vi "Data Acquisition module.vi"(3 "PortName":string, 4 "Gas Presure":dbl[unit]=80000.0 min=80000.0 max=120000.0, 5 "Run":bool=TRUE) -> (0 "Pre Evaporation Water Flow Detected by sensor":dbl[unit], 1 "Flow Evaporation Water Detected by sensor":dbl[unit], 2 "MFRHA\nMass Flow Rate of Humid Air \nof Input(Kg/s)":dbl[unit])   [LabVIEW 2018]
panel:
  out "Temp Evaporator Water  Out":dbl[unit]
  out "Voltage Level FlowMeter Air ZeroFlow":dbl
  out "Voltage Level FlowMeter.Pre.EVA Ziro Flow Water":dbl
  out "Voltage Level FlowMeter.EVA ZiroFlow Water":dbl
  out "Humidity 3rd":dbl
  out "Humidity Evaporator IN":dbl
  out "Humidity Evaporator OUT":dbl
  out "Temp 3rd Air":dbl[unit]
  out "Temp Evaporator Air IN":dbl[unit]
  out "Temp Evaporator Air OUT":dbl[unit]
  out "Voltage Level Flowmeter Air":dbl
  out "Voltage Level Flowmeter.Pre Eva Water":dbl
  out "Voltage Level Flowmeter.EVA Water":dbl
  out "Temp water  Series 2":dbl[unit]
  out "Temp Pre Eva  Water OUT":dbl[unit]
  out "Temp Pre Eva water IN":dbl[unit]
  out "Temp Evaporator Water IN":dbl[unit]
  out "SHT/H":dbl[](array[numeric])
  out "SHT/T":dbl[unit][](array[numeric])
  out "EEP":dbl[](array[numeric])
  out "MPX":dbl[](array[numeric])
  out "DS18b20":dbl[unit][](array[numeric])
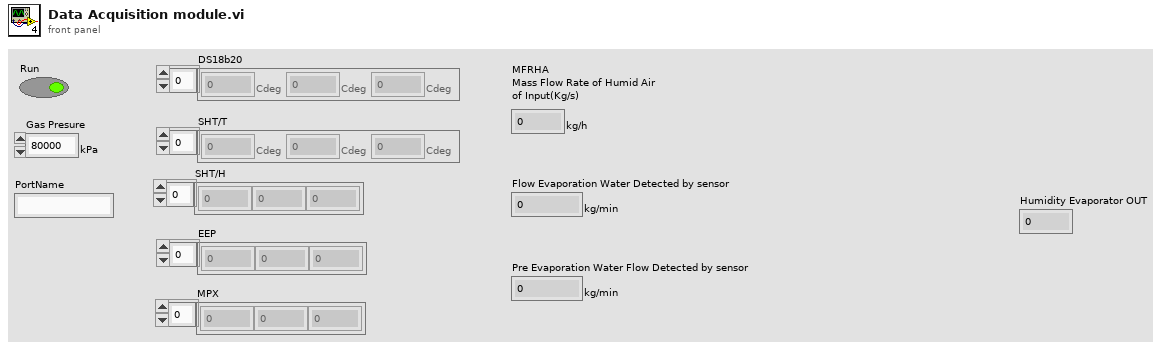
[diagram p1: front panel]
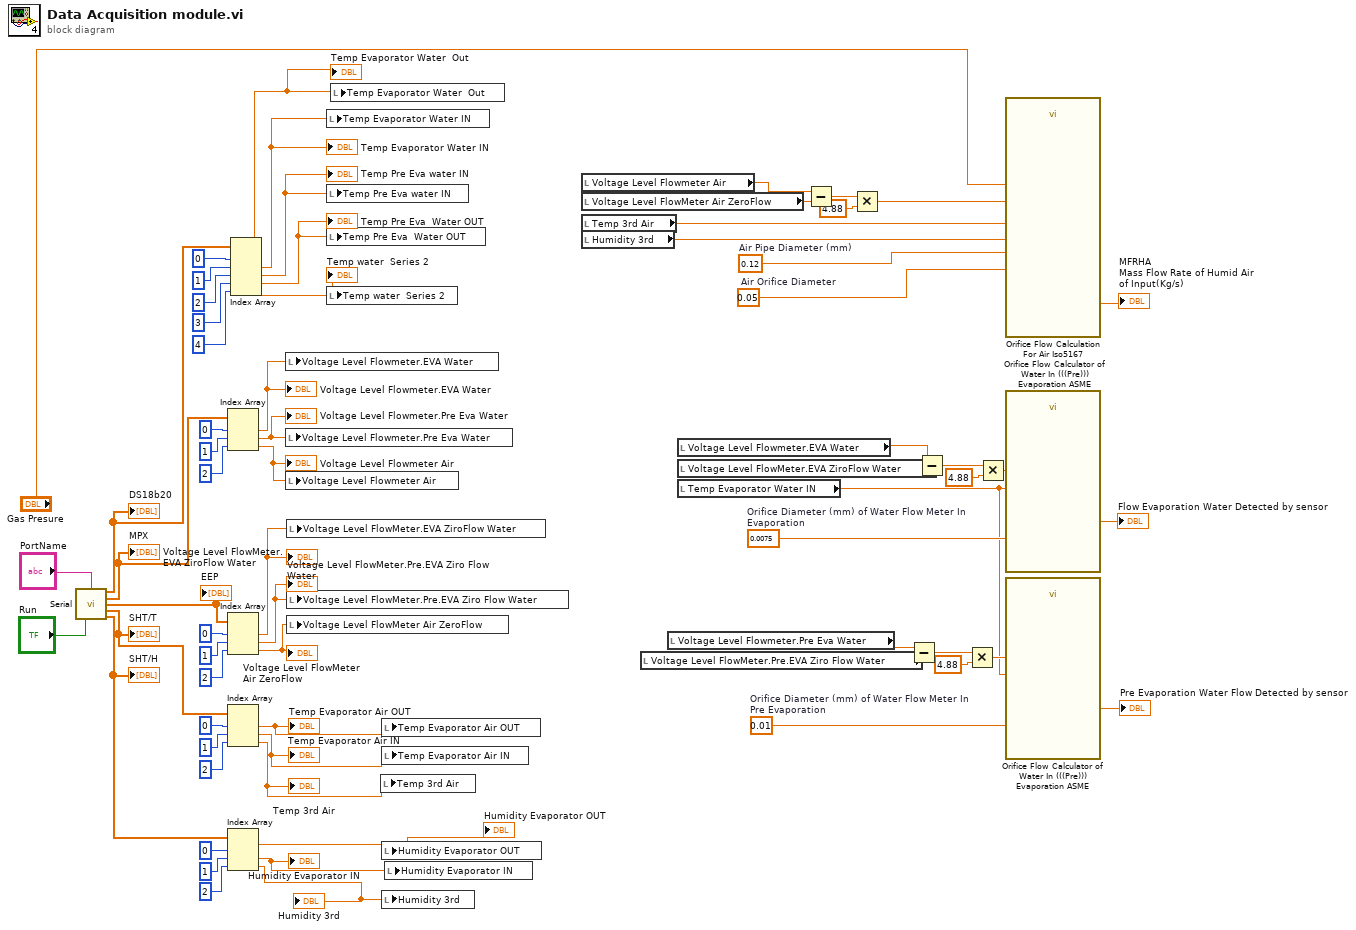
[diagram p0: block diagram]
diagram:
  w55 = dbl[unit] 0.0075  # Orifice Diameter (mm) of Water Flow Meter In Evaporation
  w66 = dbl[unit] 0.12  # Air Pipe Diameter (mm)
  w15 = dbl[unit] 0.05  # Air Orifice Diameter
  w59 = dbl[unit] 0.01  # Orifice Diameter (mm) of Water Flow Meter In Pre Evaporation
  n1 = call "Serial.vi"("PortName"="PortName", "Run"="Run") -> ("DS18b20"=w54:dbl[unit][], "MPX"=w48:dbl[], "EEP"=w33:dbl[], "SHT/H"=w44:dbl[unit][], "SHT/T"=w34:dbl[])  [unwired: 4 in, 5 out]
  "DS18b20" <- w54
  "MPX" <- w48
  "EEP" <- w33
  "SHT/T" <- w44
  "SHT/H" <- w34
  n2 = Index Array(array=w48, index #1=0 ("index"), index #2=1 ("index"), index #3=2 ("index")) -> (element #1=w29:dbl, element #2=w28:dbl, element #3=w18:dbl)
  "Voltage Level Flowmeter.EVA Water" <- w29
  "Voltage Level Flowmeter.Pre Eva Water" <- w28
  "Voltage Level Flowmeter Air" <- w18
  n3 = Index Array(array=w33, index #1=0 ("index"), index #2=1 ("index"), index #3=2 ("index")) -> (element #1=w27:dbl, element #2=w26:dbl, element #3=w25:dbl)
  "Voltage Level FlowMeter.EVA ZiroFlow Water" <- w27
  "Voltage Level FlowMeter.Pre.EVA Ziro Flow Water" <- w26
  "Voltage Level FlowMeter Air ZeroFlow" <- w25
  n4 = Index Array(array=w44, index #1=0 ("index"), index #2=1 ("index"), index #3=2 ("index")) -> (element #1=w23:dbl[unit], element #2=w24:dbl[unit], element #3=w22:dbl[unit])
  "Temp Evaporator Air OUT" <- w23
  "Temp Evaporator Air IN" <- w24
  "Temp 3rd Air" <- w22
  n5 = Index Array(array=w34, index #1=0 ("index"), index #2=1 ("index"), index #3=2 ("index")) -> (element #1=w20:dbl, element #2=w6:dbl, element #3=w21:dbl)
  "Humidity Evaporator OUT" <- w20
  "Humidity Evaporator IN" <- w6
  "Humidity 3rd" <- w21
  n6 = Index Array(array=w54, index #1=0 ("index"), index #2=1 ("index"), index #3=2 ("index"), index #4=3 ("index"), index #5=4 ("index")) -> (element #1=w3:dbl[unit], element #2=w9:dbl[unit], element #3=w37:dbl[unit], element #4=w36:dbl[unit], element #5=w35:dbl[unit])
  "Temp Evaporator Water IN" <- w9
  "Temp Pre Eva water IN" <- w37
  "Temp Pre Eva  Water OUT" <- w36
  "Temp water  Series 2" <- w35
  "Temp Evaporator Water  Out" <- w3
  n7 = local write "Voltage Level Flowmeter.EVA Water"(w29) -> ()
  n8 = local write "Voltage Level Flowmeter.Pre Eva Water"(w28) -> ()
  n9 = local write "Voltage Level Flowmeter Air"(w18) -> ()
  n10 = local write "Voltage Level FlowMeter.EVA ZiroFlow Water"(w27) -> ()
  n11 = local write "Voltage Level FlowMeter.Pre.EVA Ziro Flow Water"(w26) -> ()
  n12 = local write "Voltage Level FlowMeter Air ZeroFlow"(w25) -> ()
  n13 = local write "Temp Evaporator Water IN"(w9) -> ()
  n14 = local write "Temp Pre Eva water IN"(w37) -> ()
  n15 = local write "Temp Pre Eva  Water OUT"(w36) -> ()
  n16 = local write "Temp water  Series 2"(w35) -> ()
  n17 = local write "Temp Evaporator Water  Out"(w3) -> ()
  n18 = local write "Temp 3rd Air"(w22) -> ()
  n19 = local write "Temp Evaporator Air OUT"(w23) -> ()
  n20 = local write "Temp Evaporator Air IN"(w24) -> ()
  n21 = local write "Humidity Evaporator OUT"(w20) -> ()
  n22 = local write "Humidity 3rd"(w21) -> ()
  n23 = local write "Humidity Evaporator IN"(w6) -> ()
  n24 = local read "Voltage Level Flowmeter Air"() -> (w19:dbl)
  n25 = local read "Voltage Level FlowMeter Air ZeroFlow"() -> (w17:dbl)
  n26 = local read "Temp 3rd Air"() -> (w7:dbl[unit])
  n27 = local read "Humidity 3rd"() -> (w8:dbl)
  n28 = local read "Voltage Level FlowMeter.Pre.EVA Ziro Flow Water"() -> (w13:dbl)
  n29 = local read "Voltage Level Flowmeter.Pre Eva Water"() -> (w14:dbl)
  n30 = local read "Voltage Level Flowmeter.EVA Water"() -> (w12:dbl)
  n31 = local read "Voltage Level FlowMeter.EVA ZiroFlow Water"() -> (w11:dbl)
  n32 = local read "Temp Evaporator Water IN"() -> (w10:dbl[unit])
  n33 = Subtract(x=w19, y=w17) -> (x-y=w64:dbl)
  n34 = Multiply(x=w64, y=dbl[unit] 4.88) -> (x*y=w67:dbl[unit])
  n35 = Subtract(x=w14, y=w13) -> (x-y=w61:dbl)
  n36 = Subtract(x=w12, y=w11) -> (x-y=w57:dbl)
  n37 = Multiply(x=w61, y=dbl[unit] 4.88) -> (x*y=w60:dbl[unit])
  n38 = Multiply(x=w57, y=dbl[unit] 4.88) -> (x*y=w56:dbl[unit])
  n39 = call "Orifice Flow Calculation For Air Iso5167.vi"("RH"=w8, "Orifice Diameter"=w15, "Gas Temperature"=w7, "P1\n(Presure After Fan &\n before Orifice)"="Gas Presure", "Pipe Diameter (mm)"=w66, "Delta P\n(Presure Made By Orifice)"=w67) -> ("Mass Flow (Orifice) (Kg/h)"=→"MFRHA\nMass Flow Rate of Humid Air \nof Input(Kg/s)":dbl[unit])  [unwired: 2 out]
  n40 = call "Orifice Flow Calculator of Water In (((Pre))) Evaporation ASME.vi"("Water Temperature"=w10, "Delta P\n(Presure Made By Orifice)"=w56, "Orifice Diameter"=w55) -> ("Mass Flow (Orifice) (Kg/min)"=→"Flow Evaporation Water Detected by sensor":dbl[unit])  [unwired: 1 in, 2 out]
  n41 = call "Orifice Flow Calculator of Water In (((Pre))) Evaporation ASME.vi"("Water Temperature"=w10, "Delta P\n(Presure Made By Orifice)"=w60, "Orifice Diameter"=w59) -> ("Mass Flow (Orifice) (Kg/min)"=→"Pre Evaporation Water Flow Detected by sensor":dbl[unit])  [unwired: 1 in, 2 out]
